vi "Set Configuration.vi"(8 "error in (no error)":errorcluster, 11 "Numeric Indicator in":refnum<class "Numeric Indicator.lvclass">) -> (0 "error out":errorcluster, 3 "Numeric Indicator out":refnum<class "Numeric Indicator.lvclass">)   [LabVIEW 2015, in "Numeric Indicator.lvclass"]
uses:
  Numeric Indicator.lvclass
  IO Class/Type.ctl
  Input Signal/Input Signal.lvclass
  IO Class/IO Class.lvclass
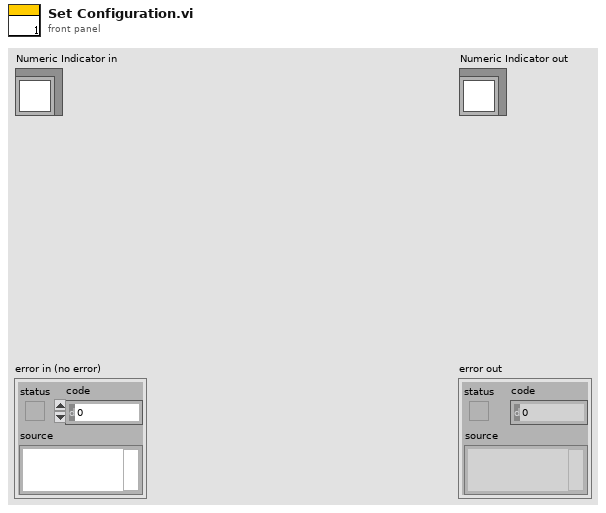
[diagram p1: front panel]
types:
  T1 = typedef "IO Class.lvclass/Type.ctl" = cluster{"Type":string}
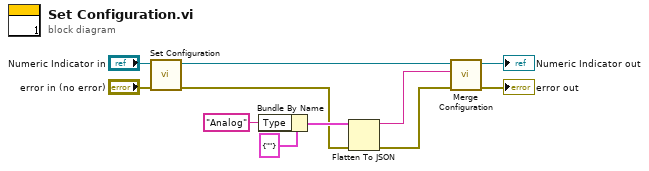
[diagram p0: block diagram]
diagram:
  n1 = call-parent "Set Configuration.vi"("error in (no error)"="error in (no error)", "Input Signal in"="Numeric Indicator in") -> ("error out"=w3:errorcluster, "Input Signal out"=w4:refnum<class "Numeric Indicator.lvclass">)  [unwired: 8 in]
  n2 = Bundle By Name(cluster=T1 {"Type"=""} ("Type"), "Type"="Analog") -> (w8:T1)
  n3 = Flatten To JSON(anything=w8, error in (no error)=w3) -> (JSON string=w7:string, 11:w6:errorcluster)  [unwired: 1 in]
  n4 = call "Merge Configuration.vi"("error in (no error)"=w6, "Additional Configuration"=w7, "IO Class in"=w4) -> ("error out"=→"error out":errorcluster, "IO Class out"=→"Numeric Indicator out":refnum<class "Numeric Indicator.lvclass">)  [unwired: 7 in]
